vi "Get Library.vi"(7 "error if not found":bool=TRUE, 8 "error in (no error)":errorcluster, 10 "library name":string, 11 "project ref":refnum<vi>) -> (0 "error out":errorcluster, 1 "found":bool, 2 "library item":refnum<vi>, 3 "project ref out":refnum<vi>)   [LabVIEW 2021, in "G Plugin Editor.lvlib"]
uses:
  G Plugin Editor.lvlib
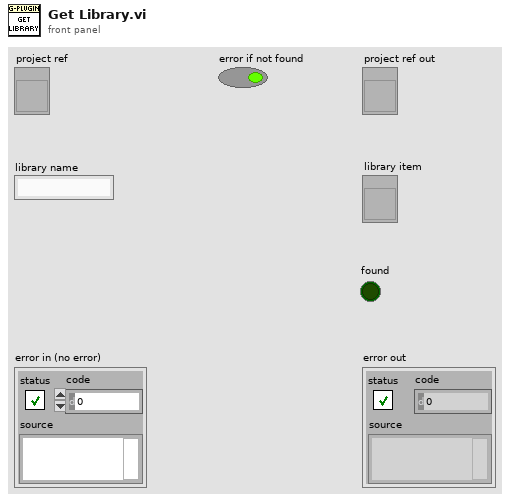
[diagram p1: front panel]
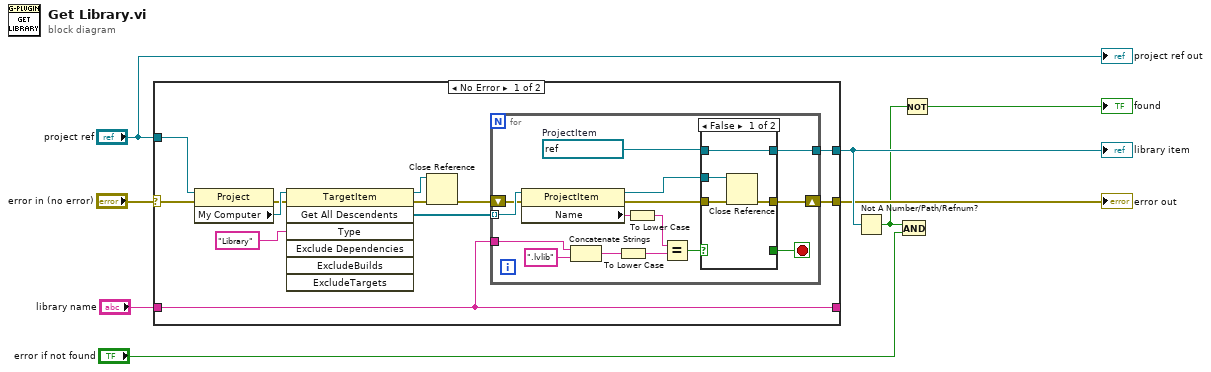
[diagram p0: block diagram]
diagram:
  n1 = case shown="No Error" "error in (no error)" {
    selector: "error in (no error)" -> [w16 w44]
    tunnel: "project ref" -> [w20 _]
    tunnel: "library name" -> [w9 w43]
    tunnel: [w15 w44] -> w4
    tunnel: [w11 _] -> w5
    tunnel: [w9 w43] -> _
    frame No Error {
      n2 = property class="Project"(reference=w20, error in=w16) -> (error out=w18:errorcluster, "My Computer"=w19:refnum<vi>)  [unwired: 1 out]
      n3 = invoke class="TargetItem" method="Get All Descendents"(reference=w19, error in=w18, "Type"="Library") -> (reference out=w13:refnum<vi>, error out=w14:errorcluster, "All Descendents"=w17:refnum<vi>[])  [unwired: 4 in, 4 out]
      n4 = Close Reference(reference=w13, error in (no error)=w14) -> (error out=w12:errorcluster)
      n5 = for {
        tunnel: w17 -> [w35] mode=indexing
        tunnel: w9 -> [w34]
        shift-right: [w28] -> w15
        shift-left: w12 -> [w32]
        tunnel: [w27] -> w11
        stop <- w22 stop-if-true
        w21 = refnum<vi> refnum  # ProjectItem
        n6 = property class="ProjectItem"(reference=w35, error in=w32) -> (reference out=w30:refnum<vi>, error out=w31:errorcluster, "Name"=w24:string)
        n7 = Concatenate Strings(w34, ".lvlib" ("string")) -> (w26:string)
        n8 = To Lower Case(string=w26) -> (all lower case string=w25:string)
        n9 = To Lower Case(string=w24) -> (all lower case string=w23:string)
        n10 = Equal?(x=w23, y=w25) -> (x = y?=w29:bool)
        n11 = case shown="False" w29 {
          selector: w29 -> [_ w40]
          tunnel: w31 -> [w39 w42]
          tunnel: w30 -> [w36 w41]
          tunnel: [w38 w42] -> w28
          tunnel: [w37 w41] -> w27
          tunnel: w21 -> [w37 _]
          tunnel: [_ w40] -> w22
          frame False {
            n12 = Close Reference(reference=w36, error in (no error)=w39) -> (error out=w38:errorcluster)
          }
          frame True {
          }
        }
      }
    }
    frame Error {
    }
  }
  "error out" <- w4
  "library item" <- w5
  n13 = Not A Number/Path/Refnum?(number/path/refnum=w5) -> (NaN/Path/Refnum?=w2:bool)
  n14 = And(x=w2, y="error if not found") -> ()  [unwired: 1 out]
  n15 = Not(x=w2) -> (.not. x?=→"found":bool)
  "project ref out" <- "project ref"
